vi "Main.vi"() -> ()   [LabVIEW 2020]
uses:
  TDefs/FP Items Properties.ctl
  TDefs/Single File Properties.ctl
  TDefs/Selected FP Items.ctl
  d6f3fa87-f68a-40a1-87be-e0999a112171.vi
  da62ed5a-17ba-4148-b1be-8aff915dfb65.vi
panel:
  in  "FP Items Properties Selected":T1
  in  "File Properties OUT":T2
  out "File Properties":T2
  out "FP Items Properties":T1
  in  "All / Selected by Name":bool
  in  "Same Desc":bool
  in  "Copy Descs to Tags":bool
  in  "PREV":bool
  in  "NEXT":bool
  out "filenames":string[](array[string])
  in  "Read entire Folder":bool
  in  "path":path
  in  "stop":bool
  in  "SAVE":bool
  in  "Copy Desc&Tags":bool
  in  "Same File":bool
  out "found index":i32[](array[numeric])
  in  "Copy VI Descr W":bool
  in  "Generate Help Tag W":bool
  in  "Copy Help Tag":bool
  in  "Copy CHM path":bool
  in  "Write":bool
  in  "Read":bool
  in  "R vi path":path
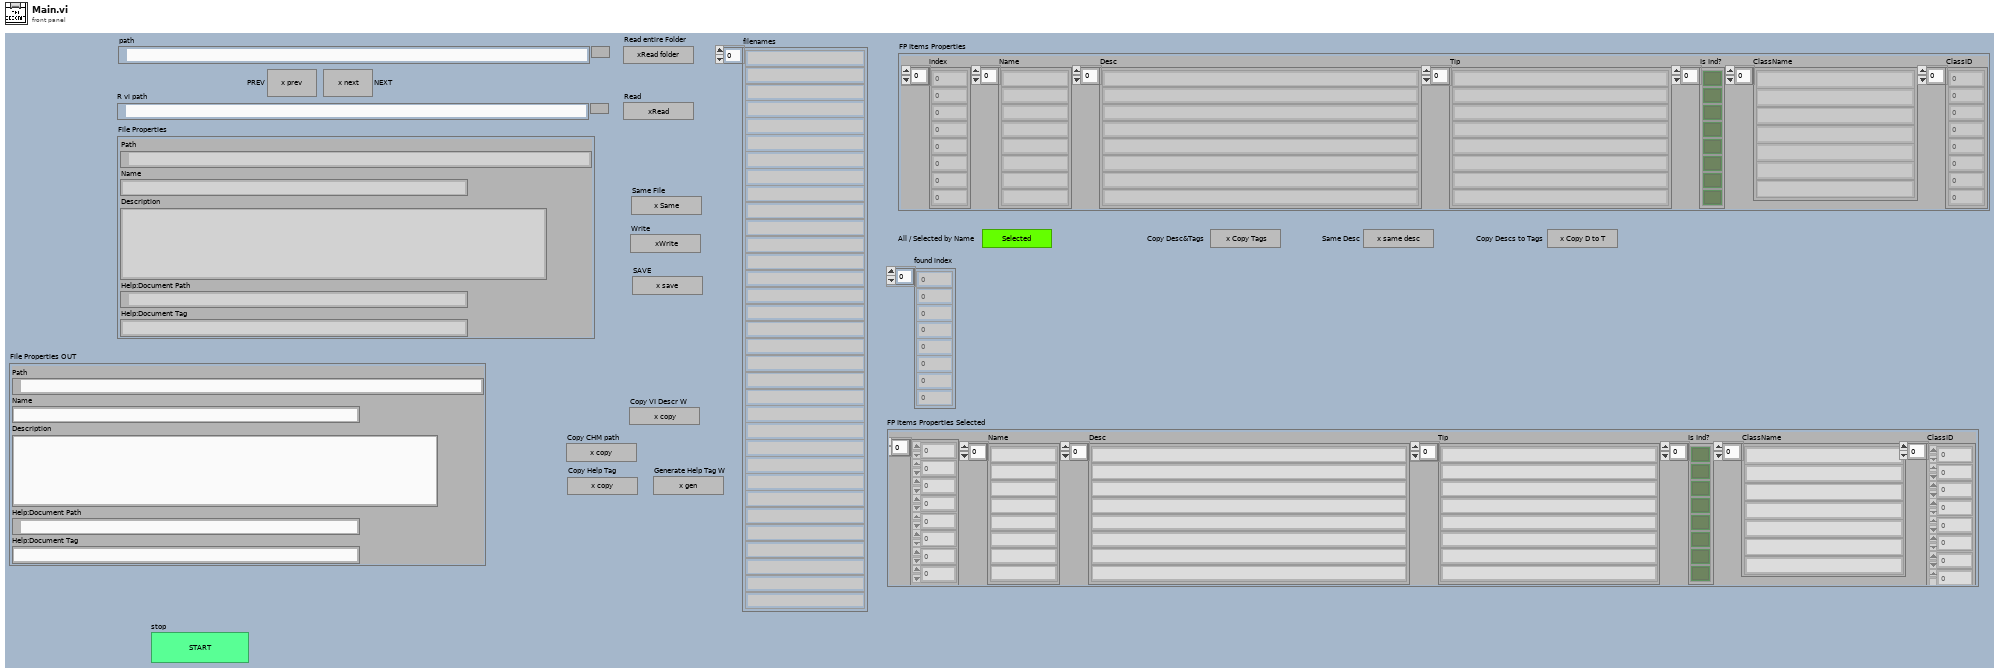
[diagram p1: front panel]
types:
  T1 = typedef "FP Items Properties.ctl" = cluster{"index":i32[], "Name":string[], "Desc":string[], "Tip":string[], "Is Ind?":bool[], "ClassName":string[], "ClassID":u32[]}
  T2 = typedef "Single File Properties.ctl" = cluster{"Path":path, "Name":string, "Description":string, "Help:Document Path":path, "Help:Document Tag":string}
  T3 = typedef "Selected FP Items.ctl" = cluster{"Names":string[], "found index":i32[]}
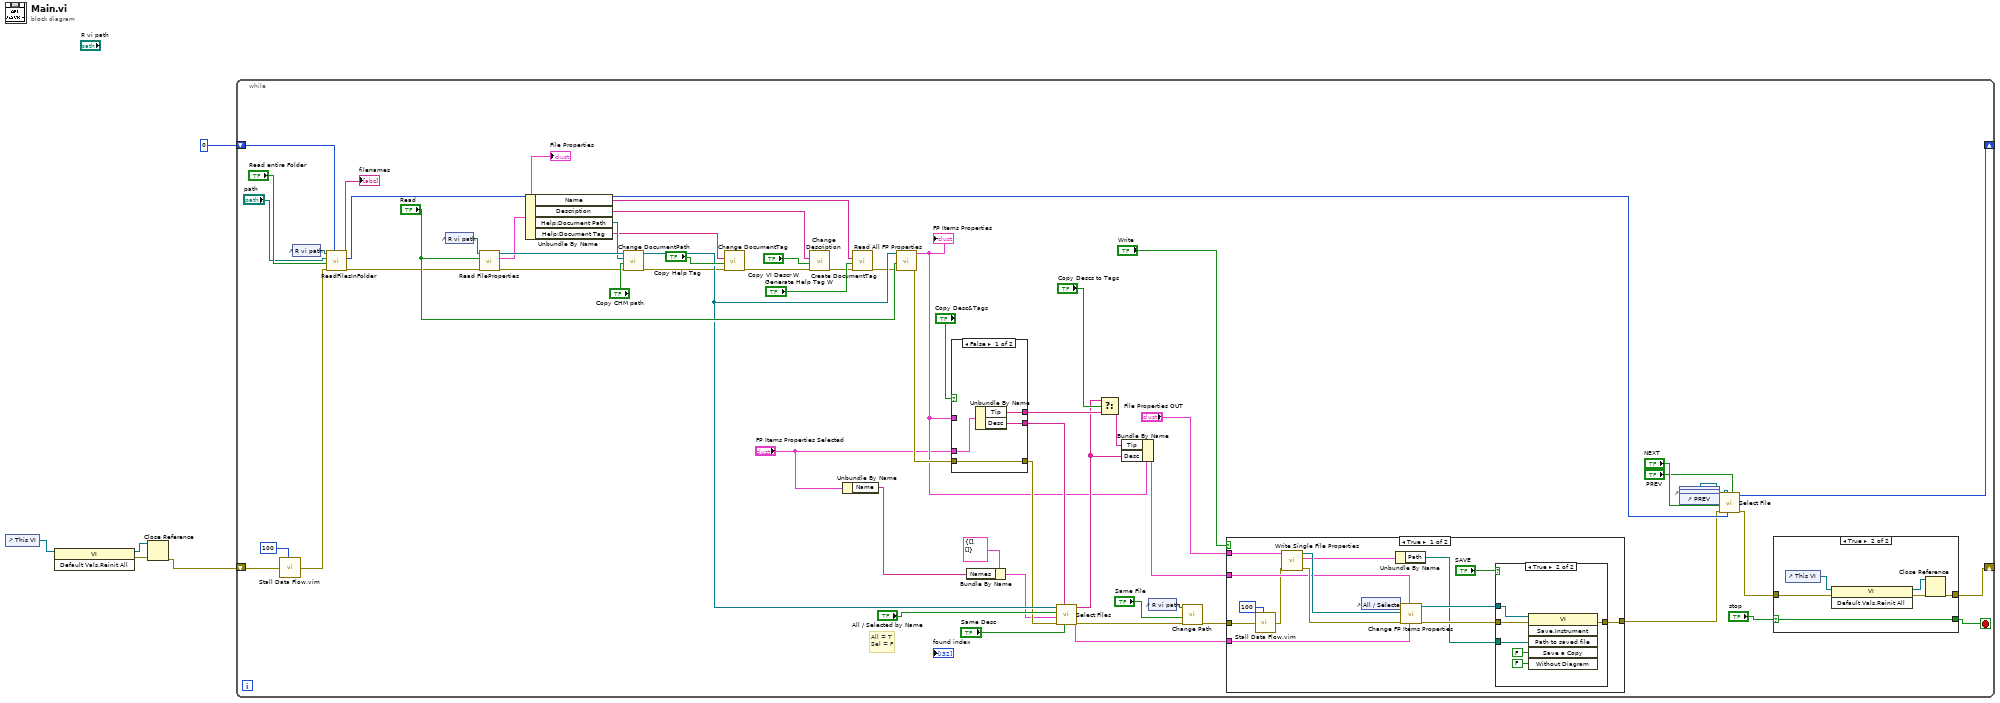
[diagram p0: block diagram]
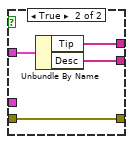
[diagram p5: hidden frame]
diagram:
  n1 = control-ref of="This VI"() -> (w4:refnum<vi>)
  n2 = invoke class="VI" method="Default Vals.Reinit All"(reference=w4) -> (reference out=w2:refnum<vi>, error out=w3:errorcluster)  [unwired: 2 in, 1 out]
  n3 = Close Reference(reference=w2, error in (no error)=w3) -> (error out=w1:errorcluster)
  n4 = while {
    shift-right: [w47] -> _
    shift-left: w1 -> [w19]
    shift-right: [w66] -> _
    shift-left: 0 -> [w65]
    stop <- w49 stop-if-true
    # "All = T\nSel = F"
    n5 = call "Stall Data Flow.vim"("value in"=w19, "milliseconds to wait"=u32 100) -> ("value out"=w18:errorcluster)  [unwired: 1 out]
    n6 = control-ref of="R vi path"() -> (w34:refnum<vi>)
    n7 = call "ReadFilesInFolder.vi"("Numeric"=w65, "error in (no error)"=w18, "Read entire Folder"="Read entire Folder", "path"="path", "Path in"=w34) -> ("error out"=w53:errorcluster, "t"=w64:i32, "filenames"=→"filenames":string[])  [unwired: 4 in]
    n8 = control-ref of="R vi path"() -> (w33:refnum<vi>)
    n9 = call "Read FileProperties.vi"("error in (no error)"=w53, "Read"="Read", "Path in"=w33) -> ("error out"=w43:errorcluster, "File Properties"=w12:T2, "VI out"=w51:refnum<vi>)  [unwired: 6 in]
    "File Properties" <- w12
    n10 = Unbundle By Name(w12) -> ("Name"=w13:string, "Description"=w14:string, "Help:Document Path"=w16:path, "Help:Document Tag"=w15:string)
    n11 = call "Change DocumentPath.vi"("error in (no error)"=w43, "Copy CHM path"="Copy CHM path", "Help.Path"=w16) -> ("error out"=w42:errorcluster)  [unwired: 8 in]
    n12 = call "Change DocumentTag.vi"("error in (no error)"=w42, "Copy Help Tag"="Copy Help Tag", "Help.Tag"=w15) -> ("error out"=w41:errorcluster)  [unwired: 8 in]
    n13 = call "Change Description.vi"("error in (no error)"=w41, "Copy VI Descr W"="Copy VI Descr W", "Description"=w14) -> ("error out"=w39:errorcluster)  [unwired: 8 in]
    n14 = Unbundle By Name("FP Items Properties Selected") -> ("Name"=w6:string[])
    n15 = call "Create DocumentTag.vi"("error in (no error)"=w39, "Generate Help Tag W"="Generate Help Tag W", "Name"=w13) -> ("error out"=w40:errorcluster)  [unwired: 8 in]
    n16 = call "Read All FP Properties.vi"("error in (no error)"=w40, "Read"="Read", "VI in"=w51) -> ("error out"=w63:errorcluster, "Properties out"=w8:T1)  [unwired: 7 in]
    "FP Items Properties" <- w8
    n17 = case shown="False" "Copy Desc&Tags" {
      tunnel: w63 -> [w101 w104]
      tunnel: [w98 w103] -> w44
      tunnel: [w99 w102] -> w45
      tunnel: [w101 w104] -> w28
      tunnel: "FP Items Properties Selected" -> [w100 _]
      tunnel: w8 -> [_ w105]
      frame False {
        n18 = Unbundle By Name(w100) -> ("Tip"=w99:string[], "Desc"=w98:string[])
      }
      frame True {
        n19 = Unbundle By Name(w105) -> ("Tip"=w102:string[], "Desc"=w103:string[])
      }
    }
    n20 = Bundle By Name(cluster=T3 {"Names"=[], "found index"=[]} ("Select FP Item In"), "Names"=w6) -> (w10:T3)
    n21 = call "Select Files.vi"("Same Desc"="Same Desc", "Desc in"=w44, "error in (no error)"=w28, "Select FP Item In"=w10, "All / Selected by Name"="All / Selected by Name", "VI in"=w51) -> ("error out"=w27:errorcluster, "Select FP Item Out"=w9:T3, "Desc out"=w31:string[])  [unwired: 3 in]
    n22 = Select(t=w31, s="Copy Descs to Tags", f=w45) -> (s? t:f=w32:string[])
    n23 = Bundle By Name(cluster=w8, "Tip"=w32, "Desc"=w31) -> (w30:T1)
    n24 = control-ref of="R vi path"() -> (w29:refnum<vi>)
    n25 = call "Change Path.vi"("error in (no error)"=w27, "Same File"="Same File", "Path in"=w29) -> ("error out"=w54:errorcluster)  [unwired: 8 in]
    n26 = case shown="True" "Write" {
      tunnel: w54 -> [w68 w89]
      tunnel: [w76 w89] -> w38
      tunnel: w30 -> [w75 _]
      tunnel: "File Properties OUT" -> [w71 _]
      tunnel: w9 -> [w67 _]
      frame True {
        n27 = call "Stall Data Flow.vim"("value in"=w68, "milliseconds to wait"=u32 100) -> ("value out"=w69:errorcluster)  [unwired: 1 out]
        n28 = call "Write Single File Properties.vi"("error in (no error)"=w69, "File Properties OUT in"=w71) -> ("error out"=w80:errorcluster, "File Properties OUT out"=w74:T2, "VI out"=w81:refnum<vi>)  [unwired: 7 in]
        n29 = control-ref of="All / Selected by Name"() -> (w72:refnum<vi>)
        n30 = Unbundle By Name(w74) -> ("Path"=w73:path)
        n31 = call "Change FP Items Properties.vi"("Select FP Item In"=w67, "Properties in"=w75, "error in (no error)"=w80, "VI in"=w81, "Boolean in"=w72) -> ("error out"=w77:errorcluster, "VI out"=w78:refnum<vi>)  [unwired: 5 in]
        n32 = case shown="True" "SAVE" {
          tunnel: w73 -> [_ w88]
          tunnel: w78 -> [_ w85]
          tunnel: w77 -> [w82 w84]
          tunnel: [w82 w83] -> w76
          frame False {
          }
          frame True {
            n33 = invoke class="VI" method="Save.Instrument"(reference=w85, error in=w84, "Path to saved file"=w88, "Save a Copy"=FALSE, "Without Diagram"=FALSE) -> (error out=w83:errorcluster)  [unwired: 1 in, 5 out]
          }
        }
      }
      frame False {
      }
    }
    n34 = control-ref of="Read entire Folder"() -> (w22:refnum<vi>)
    n35 = control-ref of="NEXT"() -> (w21:refnum<vi>)
    n36 = control-ref of="PREV"() -> (w20:refnum<vi>)
    n37 = call "Select File.vi"("PREV"="PREV", "t in"=w64, "Bool Refnum in"=w21, "error in (no error)"=w38, "NEXT"="NEXT", "Bool Refnum 3"=w20, "Boolean in"=w22) -> ("error out"=w48:errorcluster, "t out"=w66:i32)  [unwired: 3 in]
    n38 = case shown="True" "stop" {
      selector: "stop" -> [w91 w94]
      tunnel: [w91 w94] -> w49
      tunnel: w48 -> [w90 w93]
      tunnel: [w90 w92] -> w47
      frame False {
      }
      frame True {
        n39 = control-ref of="This VI"() -> (w97:refnum<vi>)
        n40 = invoke class="VI" method="Default Vals.Reinit All"(reference=w97, error in=w93) -> (reference out=w95:refnum<vi>, error out=w96:errorcluster)  [unwired: 1 in, 1 out]
        n41 = Close Reference(reference=w95, error in (no error)=w96) -> (error out=w92:errorcluster)
      }
    }
  }
